vi "Test.vi"   [LabVIEW 2012]
doc: "This VI is called when test mode begins, and will automatically be terminated when it ends. You can add manual or automatic tests and invoke them from the dashboard."
uses:
  Robot Global Data.vi
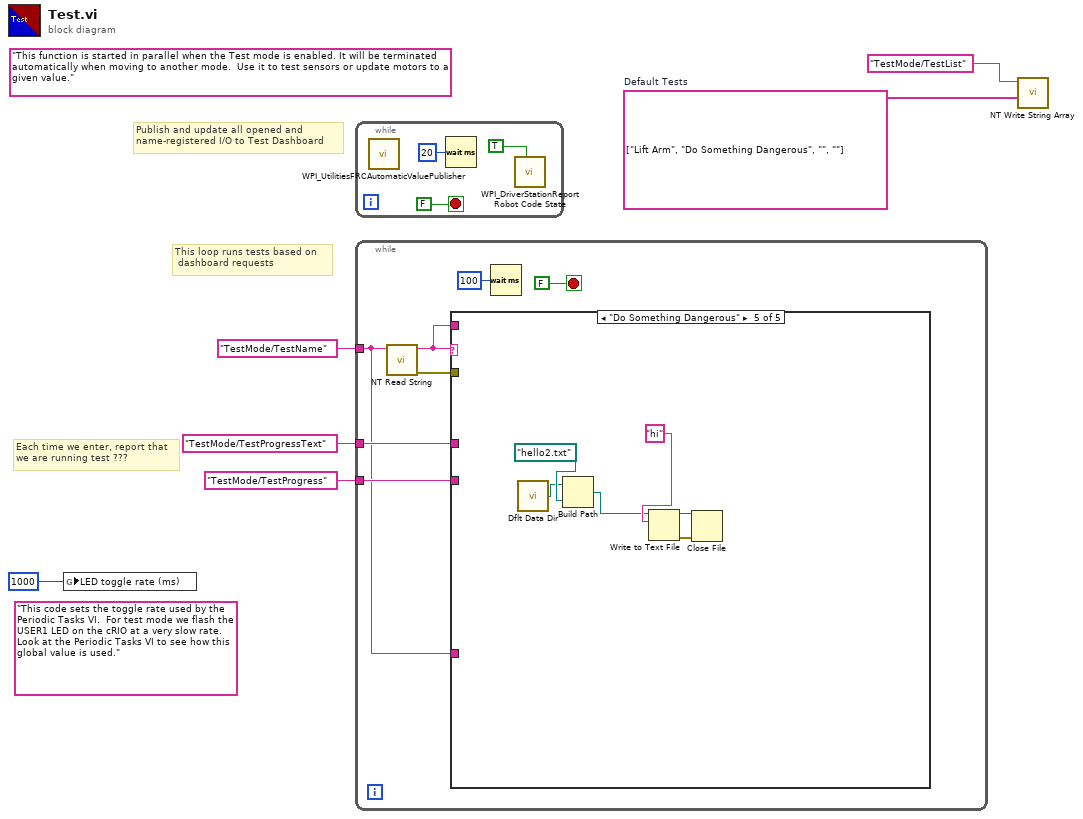
[diagram p0: block diagram]
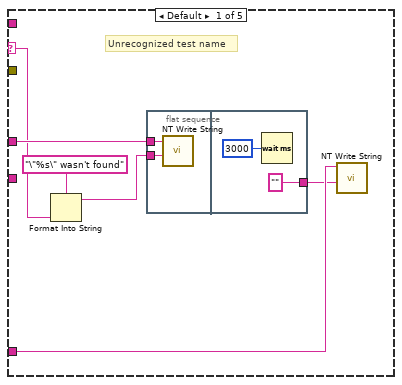
[diagram p2: hidden frame]
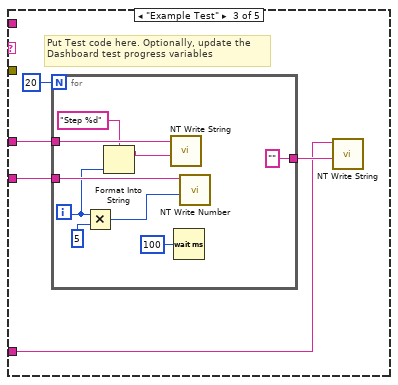
[diagram p4: hidden frame]
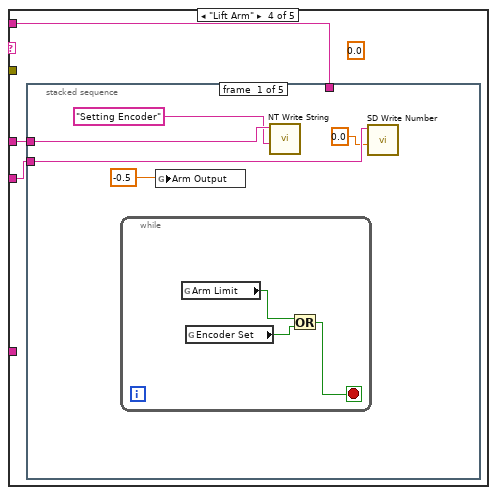
[diagram p5: hidden frame]
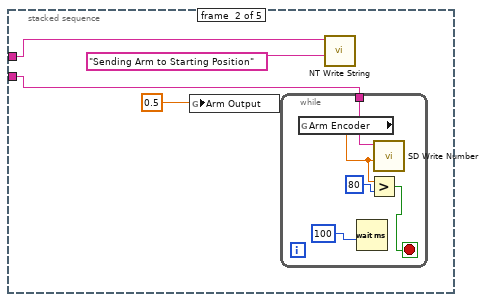
[diagram p6: hidden frame]
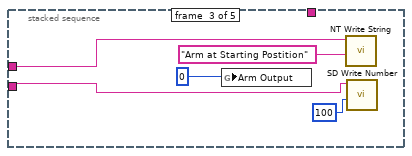
[diagram p7: hidden frame]
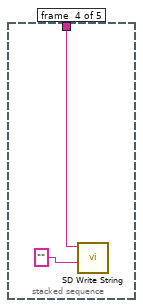
[diagram p8: hidden frame]
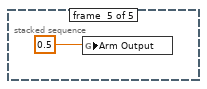
[diagram p9: hidden frame]
diagram:
  w2 = string[] ["Lift Arm", "Do Something Dangerous", "", ""]  # Default Tests
  (unwired) "This code sets the toggle rate used by the Periodic Tasks VI.  For test mode we flash the USER1 LED on the cRIO at a very slow rate.  Look at the Periodic Tasks VI to see how this global value is used."
  (unwired) "This function is started in parallel when the Test mode is enabled. It will be terminated automatically when moving to another mode.  Use it to test sensors or update motors to a given value."
  # "This loop runs tests based on \n dashboard requests"
  # "Publish and update all opened and\nname-registered I/O to Test Dashboard"
  # "Each time we enter, report that\nwe are running test ???"
  n1 = global write "Robot Global Data.vi" "LED toggle rate (ms)"(u32 1000 ("LED ms toggle rate")) -> ()
  n2 = while {
    stop <- FALSE stop-if-true
    n3 = call <vilib>:"WPI_UtilitiesFRCAutomaticValuePublisher.vi"() -> ()  [unwired: 12 in]
    n4 = Wait (ms)(milliseconds to wait=u32 20) -> ()  [unwired: 1 out]
    n5 = call <vilib>:"WPI_DriverStationReport Robot Code State.vi"("Test"=TRUE ("Autonomous")) -> ()  [unwired: 10 in, 1 out]
  }
  n6 = while {
    tunnel: "TestMode/TestName" ("Name") -> [w11]
    tunnel: "TestMode/TestProgressText" ("Name") -> [w14]
    tunnel: "TestMode/TestProgress" ("Name") -> [w13]
    stop <- FALSE stop-if-true
    n7 = call <vilib>:"NT Read String.vi"("Name"=w11) -> ("error out"=w10:errorcluster, "String"=w12:string)  [unwired: 9 in]
    n8 = case shown="\"Do Something Dangerous\"" w12 {
      selector: w12 -> [w21 _ _ _ _]
      tunnel: w11 -> [w18 _ w27 _ _]
      tunnel: w14 -> [w22 _ w30 w43 _]
      tunnel: w13 -> [_ _ w31 w41 _]
      tunnel: w12 -> [_ _ _ w42 _]
      tunnel: w10 -> [_ _ _ _ _]
      frame Default {
        # "Unrecognized test name"
        n9 = Format Into String(format string="\"%s\" wasn't found" ("Name"), w21) -> (resulting string=w20:string)  [unwired: 2 in, 1 out]
        n10 = flat-sequence {
          tunnel: w22 -> [w23]
          tunnel: w20 -> [w24]
          tunnel: ["" ("Name")] -> w17
          frame #0 {
            n11 = call <vilib>:"NT Write String.vi"("String"=w24, "Name"=w23) -> ()  [unwired: 9 in, 1 out]
          }
          frame #1 {
            n12 = Wait (ms)(milliseconds to wait=u32 3000) -> ()  [unwired: 1 out]
          }
        }
        n13 = call <vilib>:"NT Write String.vi"("String"=w17, "Name"=w18) -> ()  [unwired: 9 in, 1 out]
      }
      frame "" {
        # "No test to run"
      }
      frame "Example Test" {
        # "Put Test code here. Optionally, update the\nDashboard test progress variables"
        n14 = for {
          N: 20 -> [_]
          tunnel: w31 -> [w40]
          tunnel: w30 -> [w38]
          tunnel: ["" ("String")] -> w28
          i -> [w35]
          n15 = Multiply(x=w35, y=u32 5 ("milliseconds to wait")) -> (x*y=w36:u32)
          n16 = Format Into String(format string="Step %d", w35) -> (resulting string=w33:string)  [unwired: 2 in, 1 out]
          n17 = call <vilib>:"NT Write String.vi"("String"=w33, "Name"=w38) -> ()  [unwired: 9 in, 1 out]
          n18 = Wait (ms)(milliseconds to wait=u32 100) -> ()  [unwired: 1 out]
          n19 = call <vilib>:"NT Write Number.vi"("Numeric"=w36, "Name"=w40) -> ()  [unwired: 9 in, 1 out]
        }
        n20 = call <vilib>:"NT Write String.vi"("String"=w28, "Name"=w27) -> ()  [unwired: 9 in, 1 out]
      }
      frame "Lift Arm" {
        (unwired) 0.0
        n21 = stacked-sequence {
          tunnel: w43 -> [w48 w53 w64 _ _]
          tunnel: w42 -> [_ _ _ w67 _]
          tunnel: w41 -> [w45 w54 w63 _ _]
          frame #0 {
            n22 = while {
              stop <- w49 stop-if-true
              n23 = global read "Robot Global Data.vi" "Arm Limit"() -> (w50:bool)
              n24 = global read "Robot Global Data.vi" "Encoder Set"() -> (w51:bool)
              n25 = Or(x=w50, y=w51) -> (x .or. y?=w49:bool)
            }
            n26 = global write "Robot Global Data.vi" "Arm Output"(-0.5) -> ()
            n27 = call <vilib>:"NT Write String.vi"("String"="Setting Encoder", "Name"=w48) -> ()  [unwired: 9 in, 1 out]
            n28 = call <vilib>:"SD Write Number.vi"("Numeric"=0.0, "Name"=w45) -> ()  [unwired: 8 in, 2 out]
          }
          frame #1 {
            n29 = global write "Robot Global Data.vi" "Arm Output"(0.5) -> ()
            n30 = while {
              tunnel: w54 -> [w60]
              stop <- w56 stop-if-true
              n31 = global read "Robot Global Data.vi" "Arm Encoder"() -> (w58:dbl)
              n32 = Wait (ms)(milliseconds to wait=100) -> ()  [unwired: 1 out]
              n33 = Greater?(x=w58, y=80) -> (0:w56:bool)
              n34 = call <vilib>:"SD Write Number.vi"("Numeric"=w58, "Name"=w60) -> ()  [unwired: 8 in, 2 out]
            }
            n35 = call <vilib>:"NT Write String.vi"("String"="Sending Arm to Starting Position", "Name"=w53) -> ()  [unwired: 9 in, 1 out]
          }
          frame #2 {
            n36 = global write "Robot Global Data.vi" "Arm Output"(0) -> ()
            n37 = call <vilib>:"NT Write String.vi"("String"="Arm at Starting Postition", "Name"=w64) -> ()  [unwired: 9 in, 1 out]
            n38 = call <vilib>:"SD Write Number.vi"("Numeric"=100, "Name"=w63) -> ()  [unwired: 8 in, 2 out]
          }
          frame #3 {
            n39 = call <vilib>:"SD Write String.vi"("String"="", "Name"=w67) -> ()  [unwired: 8 in, 2 out]
          }
          frame #4 {
            n40 = global write "Robot Global Data.vi" "Arm Output"(0.5) -> ()
          }
        }
      }
      frame "Do Something Dangerous" {
        n41 = call <vilib>:"Dflt Data Dir.vi"() -> ("App:Default Data Directory"=w72:path)
        n42 = Build Path(base path=w72, name or relative path=path "hello2.txt") -> (appended path=w69:path)
        n43 = Write to Text File(file (use dialog)=w69, text="hi") -> (refnum out=w70:refnum<file>, error out=w71:errorcluster)  [unwired: 2 in, 1 out]
        n44 = Close File(refnum=w70, error in=w71) -> ()  [unwired: 2 out]
      }
    }
    n45 = Wait (ms)(milliseconds to wait=u32 100) -> ()  [unwired: 1 out]
  }
  n46 = call <vilib>:"NT Write String Array.vi"("String Array"=w2, "Name"="TestMode/TestList") -> ()  [unwired: 9 in, 1 out]
